vi "ATDome_monitorCommand_stopMotionAllAxis.vi"(8 "error in (no error)":errorcluster, 11 "command_stopMotionAllAxis_Ctl":T1) -> (0 "error out":errorcluster, 2 "function return":i32, 3 "command_stopMotionAllAxis_Ctl out":T1)   [LabVIEW 2016, in "SALLV_ATDome.lvlib"]
doc: "int ATDome_shm_monitorCommand_stopMotionAllAxisLV(ATDome_command_stopMotionAllAxisLV *command_stopMotionAllAxis_Ctl );"
uses:
  SALLV_ATDome.lvlib
  DataTypes/command_stopMotionAllAxis.ctl
  SALLV_ATDome.so
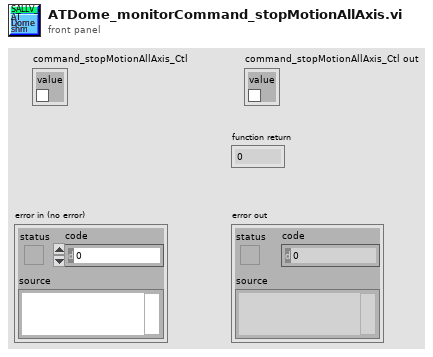
[diagram p1: front panel]
types:
  T1 = typedef "SALLV_ATDome.lvlib/command_stopMotionAllAxis.ctl" = cluster{"value":bool}
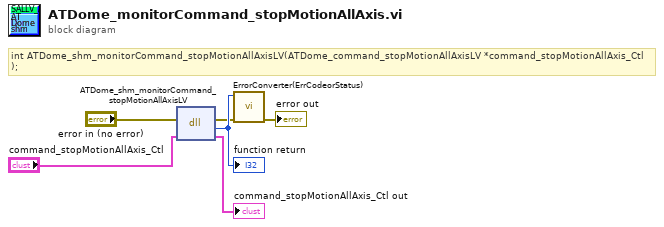
[diagram p0: block diagram]
diagram:
  # "int ATDome_shm_monitorCommand_stopMotionAllAxisLV(ATDome_command_stopMotionAllAxisLV *command_stopMotionAllAxis_Ctl );"
  n1 = dll-call lib="home/andres/Desktop/SAL_ATDome/SALLV_ATDome.*" fn="ATDome_shm_monitorCommand_stopMotionAllAxisLV"(error in="error in (no error)", "command_stopMotionAllAxis_Ctl"="command_stopMotionAllAxis_Ctl") -> (error out=w2:errorcluster, w6:i32, "command_stopMotionAllAxis_Ctl"=→"command_stopMotionAllAxis_Ctl out":T1)  [unwired: 2 in, 1 out]
  "function return" <- w6
  n2 = call "ErrorConverter(ErrCodeorStatus).vi"("error in (no error)"=w2, "error code"=w6) -> ("error out"=→"error out":errorcluster)  [unwired: 9 in]
